vi "PH_Beckhoff_PP_PU.set Trigger GUI Elements to Default.vi"(0 "i ref in":refnum<vi>, 2 "PUs":T2[](array[typedef]), 5 "error in":errorcluster) -> (14 "i ref out":refnum<vi>, 19 "error out":errorcluster)   [LabVIEW 2014, in "PH_Beckhoff_PP_PU.lvlib"]
uses:
  PH_Beckhoff_PP_PU.lvlib
  PH_PP_Common/PH_PP_Common.PUs.ctl
  PH_PP_Common/PH_PP_Common.Trigger Tags.ctl
  PH_Common/Names/PH_Names.Subsystems.ctl
  PH_PP_Common/PH_PP_Common.Devices.ctl
  PH_PP_Common/PH_PP_Common.lvlib
  PH_Common/PH_Common.lvlib
panel:
  in  "Trigger Tags":T1
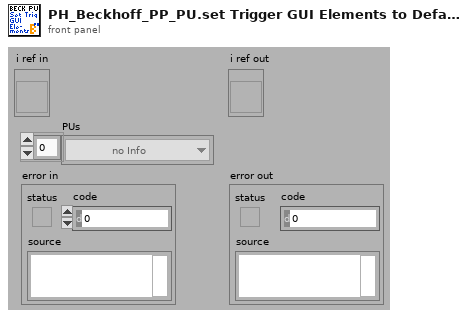
[diagram p1: front panel]
types:
  T1 = typedef "PH_PP_Common.lvlib/PH_PP_Common.Trigger Tags.ctl" = enum16{"triggered", "fired", "Status", "Last Shot"}
  T2 = typedef "PH_PP_Common.lvlib/PH_PP_Common.PUs.ctl" = enum16{"no Info", "PA-19mm-1", "PA-19mm-2", "PA-45mm-PILC", "PA-45mm-MAIN", "MA-PU-1", "MA-PU-2", "MA-PU-3", "MA-PU-4", "MA-PU-5", "MA-PU-6", "MA-FR", "MA-PILC", "PA-45mm-DP"}
  T3 = typedef "PH_Common.lvlib/PH_Names.Subsystems.ctl" = enum16{"no Info", "fs-FE", "ns-FE", "PA", "MA", "MAS", "COS", "Exp-LB", "Exp-LL", "PP", "PILS"}
  T4 = typedef "PH_Beckhoff_PP_PU.lvlib/PH_Beckhoff_PP_PU.i attribute.ctl" = cluster{"HV Meas":cluster{"Input GUI Ref":refnum<vi>, "Voltage Service ID":i32, "Voltage [V]":dbl, "Quality":bool, "# in Data":i32}[], "Trigger":cluster{"Status":cluster{"GUI Ref":refnum<vi>, "Status Service ID":i32, "Status":T5}, "last shot:":cluster{"GUI Ref":refnum<vi>, "Service ID":i32, "Time":string}, "DIs":cluster{"triggered":cluster{"GUI Ref":refnum<vi>, "# in Data":i32}, "fired":cluster{"GUI Ref":refnum<vi>, "# in Data":i32}}, "GUI Ref Indicator":refnum<vi>}[], "RR":cluster{"Status":cluster{"GUI Ref":refnum<vi>, "Status Service ID":i32, "Status":T5}, "DIs":cluster{"closed":cluster{"GUI Ref":refnum<vi>, "# in Data":i32}, "open":cluster{"GUI Ref":refnum<vi>, "# in Data":i32}}, "Close":cluster{"GUI Ref":refnum<vi>, "# in Data":i32}, "GUI Ref Indicator":refnum<vi>}[], "Igni":cluster{"Status":cluster{"GUI Ref":refnum<vi>, "Status Service ID":i32, "Status":T5}, "DIs":cluster{"heating on":cluster{"GUI Ref":refnum<vi>, "# in Data":i32}, "water on":cluster{"GUI Ref":refnum<vi>, "# in Data":i32}}, "Device on":cluster{"GUI Ref":refnum<vi>, "# in Data":i32}, "GUI Ref Indicator":refnum<vi>}[], "PSU":cluster{"Status":cluster{"GUI Ref":refnum<vi>, "Status Service ID":i32, "Status":T5}, "Limit Service ID":i32, "DIs":cluster{"inhibit":cluster{"GUI Ref":refnum<vi>, "# in Data":i32}, "end of charge":cluster{"GUI Ref":refnum<vi>, "# in Data":i32}, "HV on":cluster{"GUI Ref":refnum<vi>, "# in Data":i32}, "overtemp":cluster{"GUI Ref":refnum<vi>, "# in Data":i32}, "interlock":cluster{"GUI Ref":refnum<vi>, "# in Data":i32}, "load fault":cluster{"GUI Ref":refnum<vi>, "# in Data":i32}, "sum fault":cluster{"GUI Ref":refnum<vi>, "# in Data":i32}, "HV off":cluster{"GUI Ref":refnum<vi>, "# in Data":i32}, "DC ok":cluster{"GUI Ref":refnum<vi>, "# in Data":i32}}, "AIs":cluster{"voltage":cluster{"GUI Ref":refnum<vi>, "# in Data":i32}, "current":cluster{"GUI Ref":refnum<vi>, "# in Data":i32}}, "DAs":cluster{"inhibit":cluster{"GUI Ref":refnum<vi>, "# in Data":i32}, "interlock":cluster{"GUI Ref":refnum<vi>, "# in Data":i32}, "HV on":cluster{"GUI Ref":refnum<vi>, "# in Data":i32}, "Reset":cluster{"GUI Ref":refnum<vi>, "# in Data":i32}}, "AAs":cluster{"Voltage to set":cluster{"GUI Ref":refnum<vi>, "# in Data":i32}}, "GUI Ref Indicator":refnum<vi>}[], "reconfigured":cluster{"?":bool, "GUI Ref":refnum<vi>}, "PU Rack Type":T6, "HV Meas Info":T7, "PSU Info":T8}
  T5 = typedef "PH_StatusHandler.lvlib/PH_StatusHandler.Status.ctl" = i16
  T6 = typedef "PH_Beckhoff_PP_PU.lvlib/PH_Beckhoff_PP_PU.PU Rack Type.ctl" = enum16{"no Info", "PA 19mm", "PA 45mm", "MA PU 1 and 2", "MA PU 3 and 4", "MA PU 5 and 6", "MA FR and PILC"}
  T7 = typedef "PH_Beckhoff_PP_PU.lvlib/PH_Beckhoff_PP_PU.HV Meas Info.ctl" = cluster{"Period Time [s]":dbl, "Subtractor 1 [Hz]":dbl, "Devider 1 [Hz/kV]":dbl, "Subtractor 2 [Hz]":dbl, "Devider 2 [Hz/kV]":dbl}
  T8 = typedef "PH_Beckhoff_PP_PU.lvlib/PH_Beckhoff_PP_PU.PSU Info.ctl" = cluster{"Limits 1 [V]":cluster{"Lower":dbl, "Upper":dbl}, "Limits 2 [V]":cluster{"Lower":dbl, "Upper":dbl}}
  T9 = cluster{"Status":cluster{"GUI Ref":refnum<vi>, "Status Service ID":i32, "Status":T5}, "last shot:":cluster{"GUI Ref":refnum<vi>, "Service ID":i32, "Time":string}, "DIs":cluster{"triggered":cluster{"GUI Ref":refnum<vi>, "# in Data":i32}, "fired":cluster{"GUI Ref":refnum<vi>, "# in Data":i32}}, "GUI Ref Indicator":refnum<vi>}[]
  T10 = typedef "PH_PP_Common.lvlib/PH_PP_Common.Devices.ctl" = enum16{"no Info", "Igni", "RR", "DumpRoss", "PSU", "Trigger", "HV-Meas", "Rods", "Chiller", "Conductivity", "Mercury"}
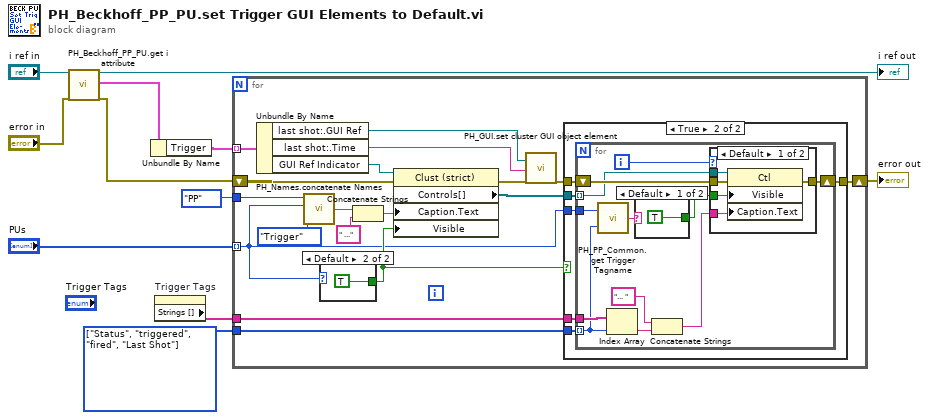
[diagram p0: block diagram]
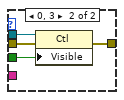
[diagram p3: hidden frame]
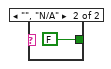
[diagram p4: hidden frame]
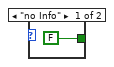
[diagram p5: hidden frame]
diagram:
  w2 = T1[] [enum."Status", enum."triggered", enum."fired", enum."Last Shot"] items=["triggered", "fired", "Status", "Last Shot"]
  n1 = call "PH_Beckhoff_PP_PU.get i attribute.vi"("i ref in"="i ref in", "error in (no error)"="error in") -> ("i ref out"=→"i ref out":refnum<vi>, "i attribute"=w9:T4, "error out"=w7:errorcluster)  [unwired: 15 in]
  n2 = Unbundle By Name(w9) -> ("Trigger"=w8:T9)
  n3 = property on="Trigger Tags" class="Enum (strict)"() -> ("Strings []"=w3:string[])  [unwired: 2 in, 2 out]
  n4 = for {
    tunnel: w8 -> [w29] mode=indexing
    shift-right: [w19] -> w10
    shift-left: w7 -> [w27]
    tunnel: "PUs" -> [w17] mode=indexing
    tunnel: w2 -> [w26]
    tunnel: w3 -> [w24]
    tunnel: PH_Names.Subsystems."PP" ("Subsystem") -> [w15]
    n5 = Unbundle By Name(w29) -> ("last shot:.GUI Ref"=w13:refnum<vi>, "last shot:.Time"=w12:string, "GUI Ref Indicator"=w25:refnum<vi>)
    n6 = call "PH_Names.concatenate Names.vi"("Devices (no info)"=PH_PP_Common.Devices."Trigger", "PU (no info)"=w17, "Subsystem"=w15) -> ("Subsystem_PU_Devices_Comm Type"=w18:string)  [unwired: 1 in]
    n7 = case shown="Default" w17 {
      tunnel: [FALSE TRUE] -> w23
      frame "no Info" {
      }
      frame Default {
      }
    }
    n8 = Concatenate Strings(w18, " ..." ("string")) -> (w21:string)
    n9 = property class="Clust (strict)"(reference=w25, error in=w27, "Caption.Text"=w21, "Visible"=w23) -> (error out=w28:errorcluster, "Controls[]"=w22:refnum<vi>[])  [unwired: 1 out]
    n10 = call "PH_GUI.set cluster GUI object element.vi"("Ctl Refnum"=w13, "Value"=w12, "error in"=w28) -> ("error out"=w14:errorcluster)  [unwired: 16 in]
    n11 = case shown="True" w23 {
      tunnel: w22 -> [_ w36]
      tunnel: w14 -> [w30 w35]
      tunnel: [w30 w34] -> w19
      tunnel: w26 -> [_ w33]
      tunnel: w17 -> [_ w32]
      tunnel: w24 -> [_ w31]
      frame False {
      }
      frame True {
        n12 = for {
          tunnel: w36 -> [w45] mode=indexing
          shift-right: [w47] -> w34
          shift-left: w35 -> [w48]
          tunnel: w32 -> [w44]
          tunnel: w33 -> [w38] mode=indexing
          tunnel: w31 -> [w46]
          i -> [w37]
          n13 = call "PH_PP_Common.get Trigger Tagname.vi"("Trigger Tag"=w38, "PU"=w44) -> ("Trigger Tagname"=w43:string)
          n14 = Index Array(array=w46, index=w38) -> (element=w41:string)
          n15 = case shown="Default" w43 {
            tunnel: [TRUE FALSE] -> w42
            frame Default {
            }
            frame "", "N/A" {
            }
          }
          n16 = Concatenate Strings("... " ("string"), w41) -> (w40:string)
          n17 = case shown="Default" w37 {
            tunnel: w48 -> [w53 w57]
            tunnel: [w52 w56] -> w47
            tunnel: w45 -> [w51 w55]
            tunnel: w42 -> [w50 w54]
            tunnel: w40 -> [w49 _]
            frame Default {
              n18 = property class="Ctl"(reference=w51, error in=w53, "Visible"=w50, "Caption.Text"=w49) -> (error out=w52:errorcluster)  [unwired: 1 out]
            }
            frame 0, 3 {
              n19 = property class="Ctl"(reference=w55, error in=w57, "Visible"=w54) -> (error out=w56:errorcluster)  [unwired: 1 out]
            }
          }
        }
      }
    }
  }
  "error out" <- w10
